vi "Position yes no done Button.vi"(8 "error in (no error)":errorcluster, 10 "Message":refnum<vi>, 11 "Button Ref":refnum<vi>) -> (0 "error out":errorcluster)   [LabVIEW 2014]
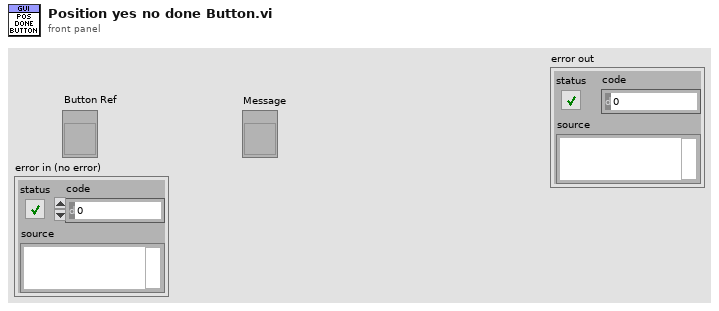
[diagram p1: front panel]
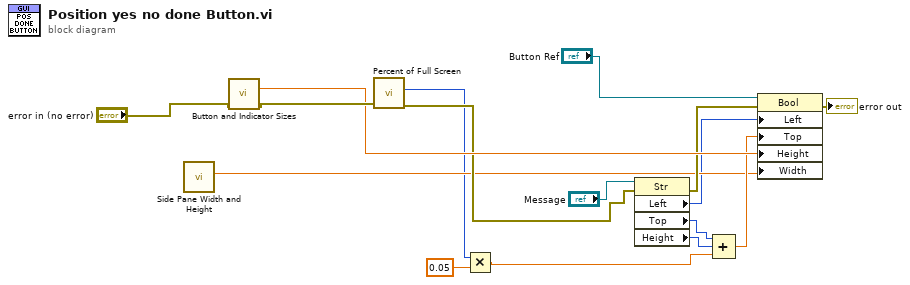
[diagram p0: block diagram]
diagram:
  n1 = call "Side Pane Width and Height.vi"() -> ("Width"=w5:dbl)  [unwired: 9 in, 2 out]
  n2 = call "Button and Indicator Sizes.vi"("error in (no error)"="error in (no error)") -> ("Button Height"=w12:dbl, "error out"=w14:errorcluster)  [unwired: 10 in, 3 out]
  n3 = call "Percent of Full Screen.vi"("error in (no error)"=w14) -> ("error out"=w10:errorcluster, "Bottom"=w4:i16)  [unwired: 8 in, 1 out]
  n4 = Multiply(x=w4, y=0.05) -> (x*y=w2:dbl)
  n5 = property class="Str"(reference="Message", error in=w10) -> (error out=w9:errorcluster, "Left"=w1:i32, "Top"=w8:i32, "Height"=w7:u32)  [unwired: 1 out]
  n6 = Compound Arithmetic op=ADD(w8, w7, w2) -> (w6:dbl)
  n7 = property class="Bool"(reference="Button Ref", error in=w9, "Left"=w1, "Top"=w6, "Height"=w12, "Width"=w5) -> (error out=→"error out":errorcluster)  [unwired: 1 out]
